vi "XCtlBlinkingLEDTask.vi"() -> ()   [LabVIEW 2012, in "XCtlBlinkingLED.xctl"]
doc: "Dynamically called VI which controls the blinking interval.\nThis VI has no external wires, its controls are set via method \"Set Ctrl Value\" from parent VI."
uses:
  XCtlBlinkingLED.xctl
panel:
  in  "BlinkingInterval":i32=100 min=100
  in  "BlinkingLED Refnum":refnum<vi>
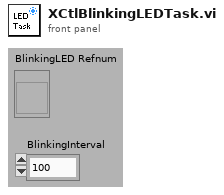
[diagram p1: front panel]
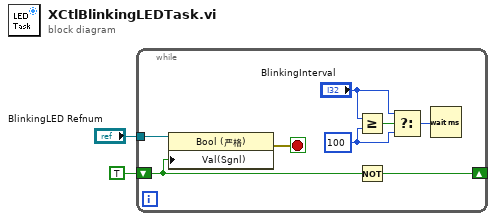
[diagram p0: block diagram]
diagram:
  n1 = while {
    shift-right: [w10] -> _
    shift-left: TRUE ("Value") -> [w8]
    tunnel: "BlinkingLED Refnum" -> [w9]
    stop <- w7 stop-if-true
    w4 = 100 ("y")
    n2 = property class="Bool (严格)"(reference=w9, "Val(Sgnl)"=w8) -> (error out=w7:errorcluster)  [unwired: 1 in, 1 out]
    n3 = Greater Or Equal?(x="BlinkingInterval", y=w4) -> (x >= y?=w5:bool)
    n4 = Not(x=w8) -> (.not. x?=w10:bool)
    n5 = Select(t="BlinkingInterval", s=w5, f=w4) -> (s? t:f=w6:i32)
    n6 = Wait (ms)(milliseconds to wait=w6) -> ()  [unwired: 1 out]
  }
